vi "脉冲编辑.vi"(8 "高速？":bool=TRUE, 11 "db file":path=path "D:/Data/波形.sqlite3") -> (3 "波形图":waveform(dbl)(graph))   [LabVIEW 2020, in "功能选择.xctl"]
uses:
  <vilib>/drjdpowell/SQLite Library/SQL Statement/SQL Statement.lvclass/SQL Statement.ctl
  <vilib>/drjdpowell/SQLite Library/SQL Connection/Open (path).vi
  <vilib>/drjdpowell/SQLite Library/SQL Statement/Bind Text.vi
  <vilib>/drjdpowell/SQLite Library/SQL Statement/First Step.vi
  <vilib>/drjdpowell/SQLite Library/SQL Statement/Column DBL.vi
  <vilib>/drjdpowell/SQLite Library/SQL Statement/Finalize (Property).vi
  <vilib>/drjdpowell/SQLite Library/SQL Connection/Open (string).vi
  <vilib>/drjdpowell/SQLite Library/SQL Statement/Step.vi
  <vilib>/drjdpowell/SQLite Library/SQL Statement/Column Type.vi
  <vilib>/drjdpowell/SQLite Library/SQL Statement/Finalize.vi
  <vilib>/AdvancedString/Path To Command Line String.vi
  <vilib>/drjdpowell/SQLite Library/SQL Connection/Execute SQL (No results).vi
  <vilib>/Utility/file.llb/Write Delimited Spreadsheet (string).vi
  <vilib>/Utility/file.llb/Read Delimited Spreadsheet (string).vi
  <vilib>/drjdpowell/SQLite Library/SQL Statement/Error Message.vi
  <vilib>/drjdpowell/SQLite Library/SQL Statement/Column String.vi
  <vilib>/drjdpowell/SQLite Library/SQL Connection/Execute SQL (1D String).vi
  <vilib>/drjdpowell/SQLite Library/SQL Connection/Connection.lvclass
  <vilib>/drjdpowell/SQLite Library/SQL Statement/SQL Statement.lvclass
  <vilib>/drjdpowell/SQLite Library/SQLite.lvlib
panel:
  in  "limit I":dbl=0.01 min=1e-08 max=3.0 format="%#_6pA"
  in  "搜索":string
  out "保存列表":i32(listbox)
  in  "脉宽":dbl=1e-05 min=5e-06 max=0.001 step=1e-06 format="%#_6ps"
  in  "脉冲电压序列":string[][](table)=[["-----end-----"]]
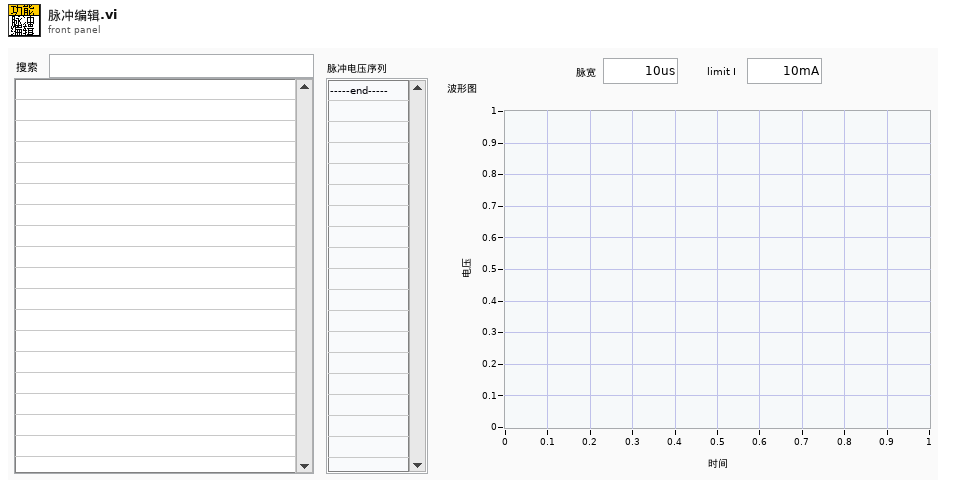
[diagram p1: front panel]
types:
  T1 = typedef "LVPoint32TypeDef.ctl" = cluster{"Horizontal":i32, "Vertical":i32}
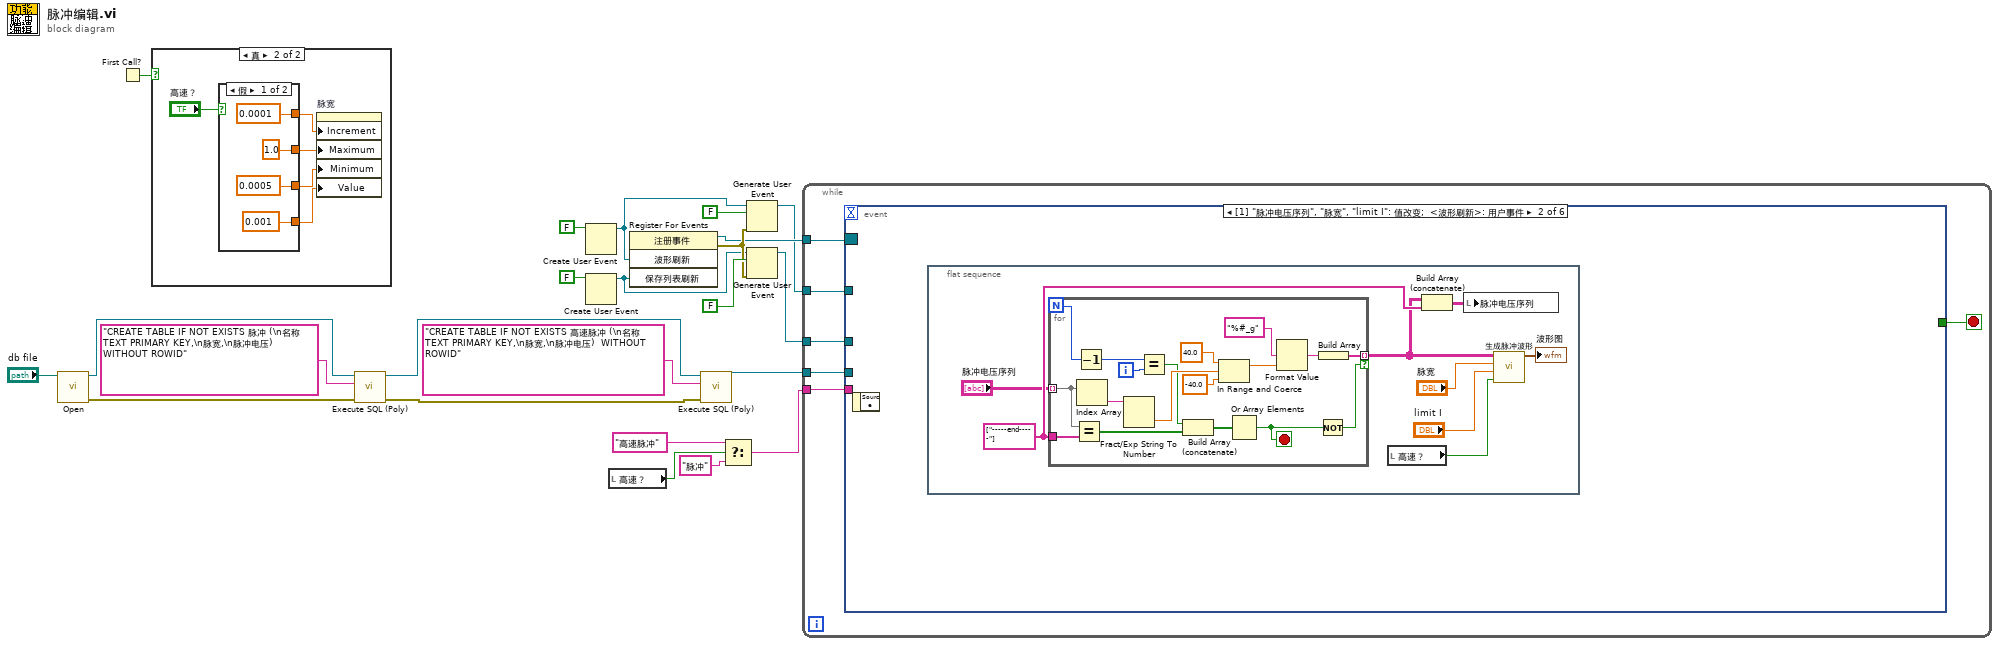
[diagram p0: block diagram]
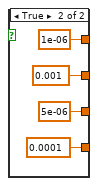
[diagram p3: hidden frame]
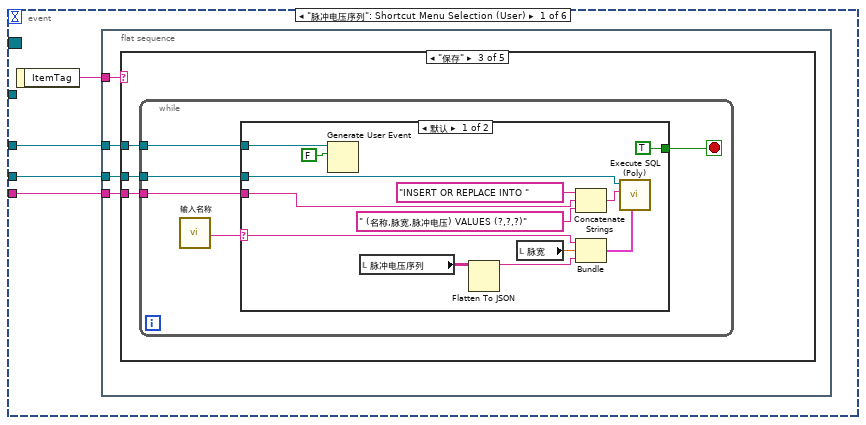
[diagram p4: hidden frame]
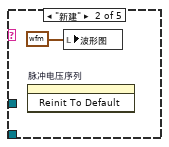
[diagram p6: hidden frame]
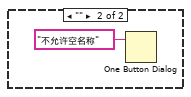
[diagram p7: hidden frame]
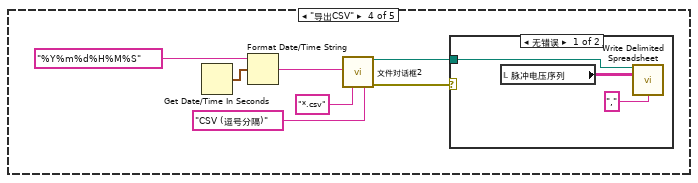
[diagram p8: hidden frame]
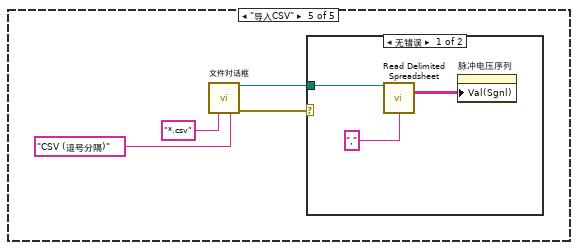
[diagram p10: hidden frame]
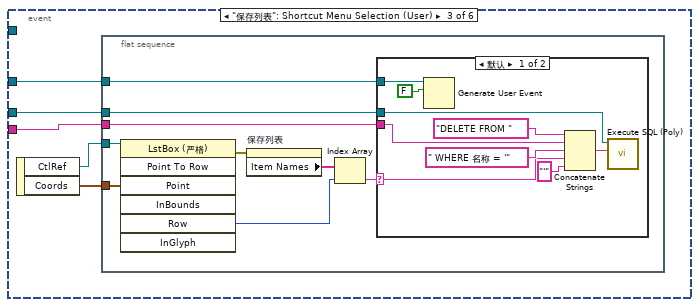
[diagram p12: hidden frame]
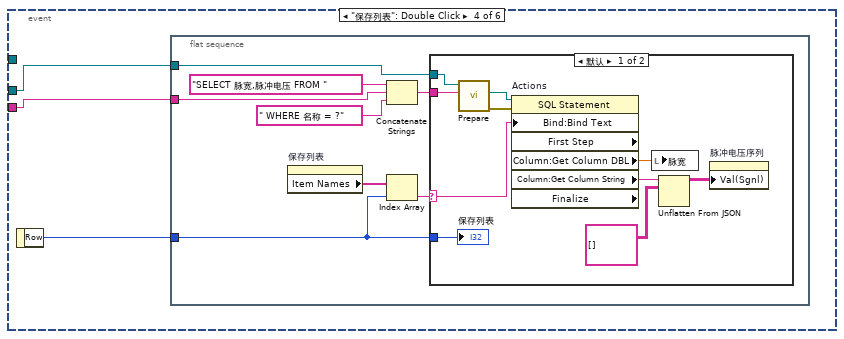
[diagram p14: hidden frame]
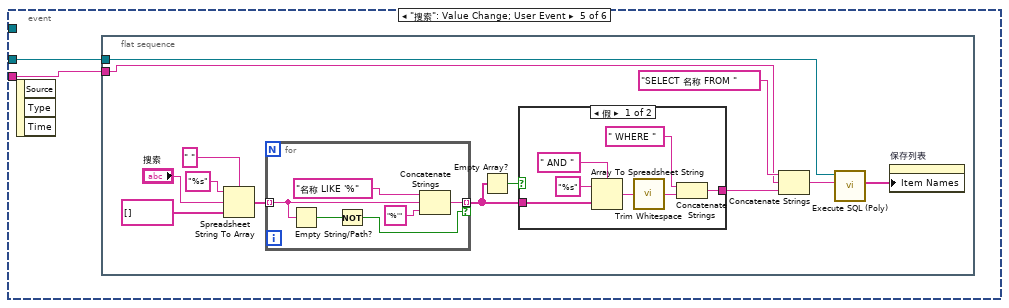
[diagram p16: hidden frame]
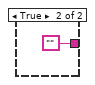
[diagram p17: hidden frame]
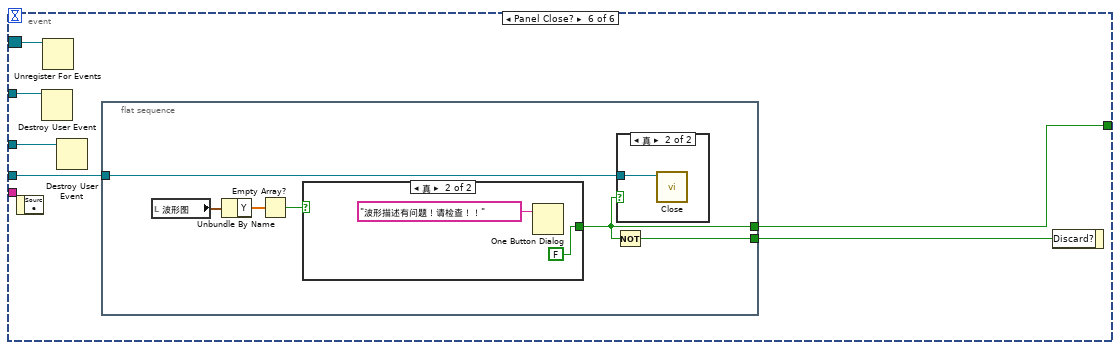
[diagram p18: hidden frame]
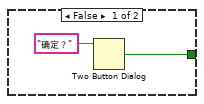
[diagram p20: hidden frame]
diagram:
  n1 = call-poly <vilib>:"Open.vi"("db file"="db file") -> ("error out"=w12:errorcluster, "SQLite Connection"=w13:refnum<class "Connection.lvclass">)  [unwired: 9 in]
  n2 = First Call?() -> (First Call?: T/F=w23:bool)
  n3 = case shown="真" w23 {
    frame False {
    }
    frame True {
      n4 = case shown="假" "高速？" {
        tunnel: [0.0005 ("数据输入界限:最小值") 5e-06 ("数据输入界限:最小值")] -> w28
        tunnel: [1.0 ("数据输入界限:最大值") 0.001 ("数据输入界限:最大值")] -> w27
        tunnel: [0.0001 ("数据输入界限:增量") 1e-06 ("数据输入界限:增量")] -> w26
        tunnel: [0.001 ("脉宽") 0.0001 ("脉宽")] -> w25
        frame False {
        }
        frame True {
        }
      }
      n5 = property on="脉宽" class="DigNum (严格)"("Increment"=w26, "Maximum"=w27, "Minimum"=w28, "Value"=w25) -> ()  [unwired: 2 in, 2 out]
    }
  }
  n6 = call-poly <vilib>:"Execute SQL (Poly).vi"("error in (no error)"=w12, "SQL"="CREATE TABLE IF NOT EXISTS 脉冲 (\n名称 TEXT PRIMARY KEY,\n脉宽,\n脉冲电压)  WITHOUT ROWID", "SQLite Connection in"=w13) -> ("error out"=w11:errorcluster, "SQLite Connection"=w10:refnum<class "Connection.lvclass">)  [unwired: 7 in]
  n7 = Create User Event(user event datatype=FALSE ("波形刷新")) -> (user event=w18:refnum<user-event>)  [unwired: 1 in, 1 out]
  n8 = Create User Event(user event datatype=FALSE ("保存列表刷新")) -> (user event=w3:refnum<user-event>)  [unwired: 1 in, 1 out]
  n9 = local read "高速？"() -> (w7:bool)
  n10 = register-events(w18, w3) -> (reference out=w16:refnum<event-registration>, error out=w17:errorcluster)  [unwired: 2 in]
  n11 = call-poly <vilib>:"Execute SQL (Poly).vi"("error in (no error)"=w11, "SQL"="CREATE TABLE IF NOT EXISTS 高速脉冲 (\n名称 TEXT PRIMARY KEY,\n脉宽,\n脉冲电压)  WITHOUT ROWID", "SQLite Connection in"=w10) -> ("SQLite Connection"=w9:refnum<class "Connection.lvclass">)  [unwired: 7 in, 1 out]
  n12 = Select(t="高速脉冲", s=w7, f="脉冲") -> (s? t:f=w4:string)
  n13 = Generate User Event(user event=w18, event data cluster=FALSE ("事件数据"), error in=w17) -> (user event out=w1:refnum<user-event>)  [unwired: 1 in, 1 out]
  n14 = Generate User Event(user event=w3, event data cluster=FALSE ("事件数据"), error in=w17) -> (user event out=w2:refnum<user-event>)  [unwired: 1 in, 1 out]
  n15 = while {
    tunnel: w16 -> [w41]
    tunnel: w9 -> [w40]
    tunnel: w2 -> [w39]
    tunnel: w4 -> [w38]
    tunnel: w1 -> [w37]
    stop <- w42 stop-if-true
    n16 = event shown="[1] \"脉冲电压序列\", \"脉宽\", \"limit I\": 值改变;  <波形刷新>: 用户事件" {
      selector: w41 -> [_ _ _ _ _ w192]
      dyn-events: _ -> [_ _ _ _ _ _]
      timeout: _ -> [_ _ _ _ _ _]
      tunnel: [_ _ _ _ _ w195] -> w42
      tunnel: w40 -> [w45 _ w118 w141 w161 w193]
      tunnel: w39 -> [w44 _ w119 _ _ w191]
      tunnel: w38 -> [w43 _ w117 w140 w162 _]
      tunnel: w37 -> [_ _ _ _ _ w190]
      event "脉冲电压序列": Shortcut Menu Selection (User) {
        n17 = event-data() -> ("ItemTag"=w46:string)  [unwired: 1 in]
        n18 = flat-sequence {
          tunnel: w46 -> [w50]
          tunnel: w45 -> [w49]
          tunnel: w44 -> [w48]
          tunnel: w43 -> [w47]
          frame #0 {
            n19 = case shown="\"保存\"" w50 {
              tunnel: w49 -> [_ _ w54 _ _]
              tunnel: w48 -> [_ _ w53 _ _]
              tunnel: w47 -> [_ _ w52 _ _]
              frame Default {
              }
              frame "新建" {
                n20 = invoke on="脉冲电压序列" class="Tbl (严格)" method="Reinit To Default"() -> ()  [unwired: 3 in, 3 out]
                n21 = local write "波形图"(waveform(dbl) {"t0"=timestamp(0 s since 1904-01-01), "dt"=1.0, "Y"=[]} ("波形图")) -> ()
              }
              frame "保存" {
                n22 = while {
                  tunnel: w54 -> [w57]
                  tunnel: w53 -> [w56]
                  tunnel: w52 -> [w55]
                  stop <- w58 stop-if-true
                  n23 = call "输入名称"() -> ("名称"=w59:string)  [unwired: 17 in, 2 out]
                  n24 = case shown="默认" w59 {
                    selector: w59 -> [w69 _]
                    tunnel: [TRUE _] -> w58
                    tunnel: w57 -> [w66 _]
                    tunnel: w56 -> [w64 _]
                    tunnel: w55 -> [w60 _]
                    frame Default {
                      n25 = Generate User Event(user event=w64, event data cluster=FALSE ("事件数据")) -> ()  [unwired: 2 in, 2 out]
                      n26 = local read "脉冲电压序列"() -> (w70:string[][])
                      n27 = Flatten To JSON(anything=w70) -> (JSON string=w71:string)  [unwired: 2 in, 1 out]
                      n28 = local read "脉宽"() -> (w72:dbl)
                      n29 = Concatenate Strings("INSERT OR REPLACE INTO " ("SQL"), w60, " (名称,脉宽,脉冲电压) VALUES (?,?,?)" ("字符串")) -> (w62:string)
                      n30 = Bundle(w69, "脉宽"=w72, "JSON string"=w71) -> (w63:cluster{string, "脉宽":dbl, "JSON string":string})  [unwired: 1 in]
                      n31 = call-poly <vilib>:"Execute SQL (Poly).vi"("Parameter(s)"=w63, "SQL"=w62, "SQLite Connection in"=w66) -> ()  [unwired: 7 in, 2 out]
                    }
                    frame "" {
                      n32 = One Button Dialog(message="不允许空名称" ("消息")) -> ()  [unwired: 1 in, 1 out]
                    }
                  }
                }
              }
              frame "导出CSV" {
                n33 = Get Date/Time In Seconds() -> (seconds since 1Jan1904=w77:timestamp)
                n34 = Format Date/Time String(time format string (%c)="%Y%m%d%H%M%S" ("时间格式字符串(%c)"), seconds (now)=w77) -> (date/time string=w76:string)  [unwired: 1 in]
                n35 = call "文件对话框2"("default name"=w76, "pattern (all files)"="*.csv" ("pattern label"), "pattern label"="CSV (逗号分隔)" ("pattern (all files)")) -> ("selected path"=w80:path, "error out"=w74:errorcluster)  [unwired: 9 in, 2 out]
                n36 = case shown="无错误" w74 {
                  tunnel: w80 -> [w83 _]
                  frame No Error {
                    n37 = local read "脉冲电压序列"() -> (w82:string[][])
                    n38 = call-poly <vilib>:"Write Delimited Spreadsheet.vi"("file path (dialog if empty)"=w83, "2D data"=w82, "delimiter (\\t)"="," ("delimiter (\\t)")) -> ()  [unwired: 11 in, 2 out]
                  }
                  frame Error {
                  }
                }
              }
              frame "导入CSV" {
                n39 = call "文件对话框"("pattern (all files)"="*.csv" ("pattern label"), "pattern label"="CSV (逗号分隔)" ("pattern (all files)")) -> ("selected path"=w87:path, "error out"=w86:errorcluster)  [unwired: 10 in, 2 out]
                n40 = case shown="无错误" w86 {
                  tunnel: w87 -> [w90 _]
                  frame No Error {
                    n41 = call-poly <vilib>:"Read Delimited Spreadsheet.vi"("file path (dialog if empty)"=w90, "delimiter (\\t)"="," ("delimiter (\\t)")) -> ("all rows"=w88:string[][])  [unwired: 8 in, 5 out]
                    n42 = property on="脉冲电压序列" class="Tbl (严格)"("Val(Sgnl)"=w88) -> ()  [unwired: 2 in, 2 out]
                  }
                  frame Error {
                  }
                }
              }
            }
          }
        }
      }
      event "脉冲电压序列", "脉宽", "limit I": Value Change; User Event {
        n43 = event-data() -> ()  [unwired: 1 in, 1 out]
        n44 = flat-sequence {
          frame #0 {
            w98 = string[] ["-----end-----"] ("电压序列")
            n45 = for {
              N -> [w108]
              tunnel: "脉冲电压序列" -> [w103] mode=indexing
              tunnel: [w111] -> w91 mode=indexing if=w99
              tunnel: w98 -> [w102]
              i -> [w107]
              stop <- w109 stop-if-true
              n46 = Equal?(x=w103, y=w102) -> (x = y?=w110:bool[])
              n47 = Decrement(x=w108) -> (x-1=w106:i32)
              n48 = Index Array(array=w103) -> (element=w116:string)  [unwired: 1 in]
              n49 = Fract/Exp String To Number(string=w116) -> (number=w112:dbl)  [unwired: 3 in, 1 out]
              n50 = Equal?(x=w106, y=w107) -> (x = y?=w104:bool)
              n51 = Build Array (concatenate)(w104, w110) -> (w105:bool[])
              n52 = In Range and Coerce(upper limit=40.0 ("上限"), x=w112, lower limit=-40.0 ("下限")) -> (coerced(x)=w100:dbl)  [unwired: 1 out]
              n53 = Or Array Elements(Boolean array=w105) -> (logical OR=w109:bool)
              n54 = Format Value(format string="%#_g" ("格式字符串"), value (0)=w100) -> (output string=w113:string)  [unwired: 1 in]
              n55 = Not(x=w109) -> (.not. x?=w99:bool)
              n56 = Build Array(w113) -> (w111:string[])
            }
            n57 = local read "高速？"() -> (w95:bool)
            n58 = Build Array (concatenate)(w91, w98) -> (w94:string[][])
            n59 = local write "脉冲电压序列"(w94) -> ()
            n60 = call "生成脉冲波形.vi"("高速？"=w95, "limit I"="limit I", "脉宽"="脉宽", "脉冲电压"=w91) -> ("波形图"=→"波形图":waveform(dbl))  [unwired: 7 in]
          }
        }
      }
      event "保存列表": Shortcut Menu Selection (User) {
        n61 = event-data() -> ("CtlRef"=w121:refnum<vi>, "Coords"=w120:T1)  [unwired: 1 in]
        n62 = flat-sequence {
          tunnel: w121 -> [w130]
          tunnel: w120 -> [w129]
          tunnel: w119 -> [w126]
          tunnel: w118 -> [w125]
          tunnel: w117 -> [w123]
          frame #0 {
            n63 = invoke class="LstBox (严格)" method="Point To Row"(reference=w130, "Point"=w129) -> (error out=w122:errorcluster, "Row"=w127:i32)  [unwired: 5 in, 5 out]
            n64 = property on="保存列表" class="LstBox (严格)"(error in=w122) -> ("Item Names"=w128:string[])  [unwired: 1 in, 2 out]
            n65 = Index Array(array=w128, index=w127) -> (element=w124:string)
            n66 = case shown="默认" w124 {
              selector: w124 -> [w137 _]
              tunnel: w125 -> [w136 _]
              tunnel: w126 -> [w134 _]
              tunnel: w123 -> [w131 _]
              frame Default {
                n67 = Generate User Event(user event=w134, event data cluster=FALSE ("事件数据")) -> ()  [unwired: 2 in, 2 out]
                n68 = Concatenate Strings("DELETE FROM " ("字符串"), w131, " WHERE 名称 = '" ("condition"), w137, "'" ("字符串")) -> (w135:string)
                n69 = call-poly <vilib>:"Execute SQL (Poly).vi"("SQL"=w135, "SQLite Connection in"=w136) -> ()  [unwired: 8 in, 2 out]
              }
              frame "" {
              }
            }
          }
        }
      }
      event "保存列表": Double Click {
        n70 = event-data() -> ("Row"=w142:i32)  [unwired: 1 in]
        n71 = flat-sequence {
          tunnel: w142 -> [w150]
          tunnel: w141 -> [w146]
          tunnel: w140 -> [w143]
          frame #0 {
            n72 = property on="保存列表" class="LstBox (严格)"() -> ("Item Names"=w149:string[])  [unwired: 2 in, 2 out]
            n73 = Concatenate Strings("SELECT 脉宽,脉冲电压 FROM " ("SELECT  statement"), w143, " WHERE 名称 = ?" ("字符串")) -> (w145:string)
            n74 = Index Array(array=w149, index=w150) -> (element=w148:string)
            n75 = case shown="默认" w148 {
              selector: w148 -> [w154 _]
              tunnel: w150 -> [w160 _]
              tunnel: w145 -> [w156 _]
              tunnel: w146 -> [w155 _]
              frame Default {
                n76 = call <vilib>:"Prepare.vi"("SQL"=w156, "SQLite Connection in"=w155) -> ("error out"=w158:errorcluster, "SQL Statement"=w159:refnum<class "SQL Statement.lvclass">)  [unwired: 5 in, 3 out]
                n77 = property on="Actions" class="SQL Statement" props=["Bind:Bind Text", "First Step", "Column:Get Column DBL", "Column:Get Column String", "Finalize"](reference=w159, error in=w158, "Bind:Bind Text"=w154) -> ("Column:Get Column DBL"=w152:dbl, "Column:Get Column String"=w151:string)  [unwired: 4 out]
                n78 = local write "脉宽"(w152) -> ()
                n79 = Unflatten From JSON(JSON string=w151, type and defaults=string[][] []) -> (value=w153:string[][])  [unwired: 5 in, 1 out]
                n80 = property on="脉冲电压序列" class="Tbl (严格)"("Val(Sgnl)"=w153) -> ()  [unwired: 2 in, 2 out]
                "保存列表" <- w160
              }
              frame "" {
              }
            }
          }
        }
      }
      event "搜索": Value Change; User Event {
        n81 = event-data() -> ()  [unwired: 1 in, 3 out]
        n82 = flat-sequence {
          tunnel: w162 -> [w165]
          tunnel: w161 -> [w164]
          frame #0 {
            n83 = Spreadsheet String To Array(delimiter (Tab)=" " ("分隔符(Tab)"), format string="%s" ("格式字符串"), spreadsheet string="搜索", array type (2D Dbl)=string[] []) -> (array=w171:string[])
            n84 = for {
              tunnel: w171 -> [w186] mode=indexing
              tunnel: [w187] -> w170 mode=indexing if=w184
              n85 = Empty String/Path?(string/path=w186) -> (empty?=w185:bool)
              n86 = Not(x=w185) -> (.not. x?=w184:bool)
              n87 = Concatenate Strings("名称 LIKE '%" ("字符串"), w186, "%'" ("condition")) -> (w187:string)
            }
            n88 = Empty Array?(array=w170) -> (empty?=w169:bool)
            n89 = case shown="假" w169 {
              tunnel: [w178 ""] -> w166
              tunnel: w170 -> [w176 _]
              frame False {
                n90 = Array To Spreadsheet String(delimiter (Tab)=" AND " ("分隔符(Tab)"), array=w176, 3:"%s" ("格式字符串")) -> (spreadsheet string=w180:string)
                n91 = call <vilib>:"Trim Whitespace.vi"("string"=w180) -> ("trimmed string"=w179:string)  [unwired: 1 in]
                n92 = Concatenate Strings(" WHERE ", w179) -> (w178:string)
              }
              frame True {
              }
            }
            n93 = Concatenate Strings("SELECT 名称 FROM " ("SQL"), w165, w166) -> (w167:string)
            n94 = call-poly <vilib>:"Execute SQL (Poly).vi"("SQL"=w167, "SQLite Connection in"=w164) -> ("Result Set"=w163:string[])  [unwired: 6 in, 3 out]
            n95 = property on="保存列表" class="LstBox (严格)"("Item Names"=w163) -> ()  [unwired: 2 in, 2 out]
          }
        }
      }
      event Panel Close? {
        n96 = event-data() -> ()  [unwired: 1 in, 1 out]
        n97 = Destroy User Event(user event=w190) -> ()  [unwired: 1 in, 1 out]
        n98 = Unregister For Events(event registration refnum=w192) -> ()  [unwired: 1 in, 1 out]
        n99 = Destroy User Event(user event=w191) -> ()  [unwired: 1 in, 1 out]
        n100 = flat-sequence {
          tunnel: [w198] -> w195
          tunnel: [w197] -> w194
          tunnel: w193 -> [w196]
          frame #0 {
            n101 = local read "波形图"() -> (w201:waveform(dbl))
            n102 = Unbundle By Name(w201) -> ("Y"=w200:dbl[])
            n103 = Empty Array?(array=w200) -> (empty?=w199:bool)
            n104 = case shown="真" w199 {
              tunnel: [w203 FALSE ("T button?")] -> w198
              frame False {
                n105 = Two Button Dialog(message="确定？" ("消息")) -> (T button?=w203:bool)  [unwired: 2 in]
              }
              frame True {
                n106 = One Button Dialog(message="波形描述有问题！请检查！！" ("消息")) -> ()  [unwired: 1 in, 1 out]
              }
            }
            n107 = Not(x=w198) -> (.not. x?=w197:bool)
            n108 = case shown="真" w198 {
              tunnel: w196 -> [_ w202]
              frame False {
              }
              frame True {
                n109 = call-dynamic "Close.vi"("SQLite Connection in"=w202) -> ()  [unwired: 10 in, 1 out]
              }
            }
          }
        }
        n110 = event-data("Discard?"=w194) -> ()  [unwired: 1 in, 1 out]
      }
    }
  }
